vi "R.vizulis 1.vi"() -> ()   [LabVIEW 2022 SP3]
uses:
  <vilib>/Utility/file.llb/Write Delimited Spreadsheet (I64).vi
  <vilib>/Utility/file.llb/Write Delimited Spreadsheet (DBL).vi
panel:
  in  "stop":bool
  out "Waveform Chart":dynamicdata(graph)
  in  "file path (dialog if empty) 2":path
  out "Array":dbl[](array[numeric])
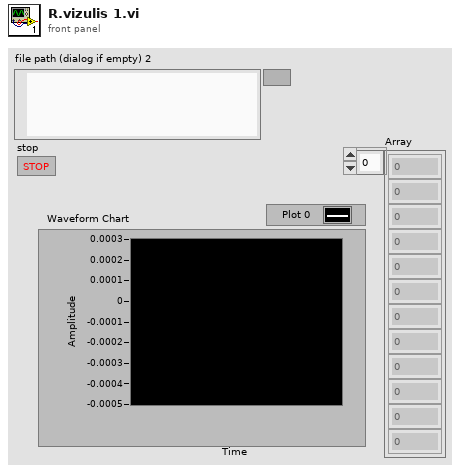
[diagram p1: front panel]
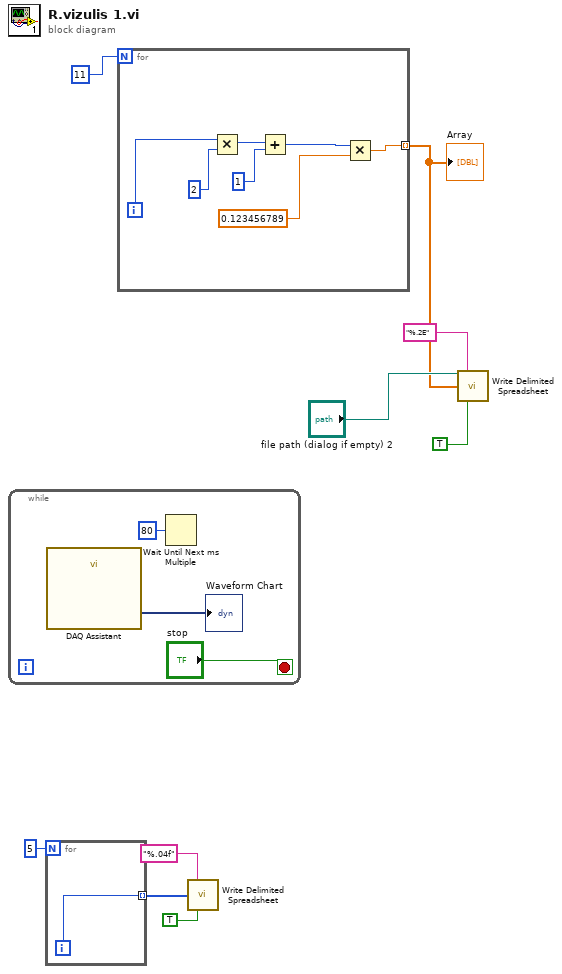
[diagram p0: block diagram]
diagram:
  n1 = while {
    stop <- "stop" stop-if-true
    n2 = call "DAQ Assistant"() -> ("data"=→"Waveform Chart":dynamicdata)  [unwired: 17 in, 2 out]
    n3 = Wait Until Next ms Multiple(millisecond multiple=u32 80) -> ()  [unwired: 1 out]
  }
  n4 = for {
    N: 5 -> [_]
    tunnel: [w13] -> w8 mode=indexing
    i -> [w13]
  }
  n5 = for {
    N: 11 -> [_]
    tunnel: [w15] -> w1 mode=indexing
    i -> [w20]
    n6 = Multiply(x=w20, y=2) -> (x*y=w18:i32)
    n7 = Add(x=w18, y=1) -> (x+y=w14:i32)
    n8 = Multiply(x=w14, y=0.123456789) -> (x*y=w15:dbl)
  }
  "Array" <- w1
  n9 = call-poly <vilib>:"Write Delimited Spreadsheet.vi"("format (%d)"="%.04f", "1D data"=w8, "transpose? (no:F)"=TRUE) -> ()  [unwired: 11 in, 2 out]
  n10 = call-poly <vilib>:"Write Delimited Spreadsheet.vi"("file path (dialog if empty)"="file path (dialog if empty) 2", "format (%.3f)"="%.2E", "1D data"=w1, "transpose? (no:F)"=TRUE) -> ()  [unwired: 10 in, 2 out]
